vi "ProgressBar-Reset specific progress bar.vi"(8 "Error in":errorcluster, 10 "Sender":enum16{"Acquisition", "Logging", "File gen"}(ring), 11 "Z-stack queue cluster":T1={"Imaging Protocol"=enum."Live Imaging", "Number of Trials"=0, "Frame Size"=512, "# Averaged frames"=0, "Dwell time (us)"=0.0, "Index of Z-plane"=0, "Timelapse?"=FALSE, "Logging process is active"=FALSE, "Speed logging enabled"=FALSE, "tdms file ref"=refnum, "path"=path "", "Trial Number"=0, "Expected # points acquired"=FALSE, "Manually stopped"=FALSE, "Ch0 data"=[], "Ch1 data"=[], "Ref Data"=[], "Last trial"=FALSE, "Ref Dwell time (us)"=0.0, "# Ref Averaged frames"=0, "Ref X Length"=0, "Ref Y Length"=0, "Points acquired"={"Ch0 last trial"=0, "Ch1 last trial"=0, "All trials"=0}} {"Ref Dwell time (us)" format="%#.6g"; "Frame Size" items=["100X100"=100, "128X128"=128, "200X200"=200, "256X256"=256, "512X512"=512, "1024x1024"=1024, "2048x2048"=2048]; "Dwell time (us)" format="%#.6g"}) -> (0 "error out":errorcluster)   [LabVIEW 2017]
uses:
  Typedefs/Logging queue element.ctl
  Typedefs/Imaging Protocols enum.ctl
  Typedefs/Frame Size.ctl
  Typedefs/Acquired points count.ctl
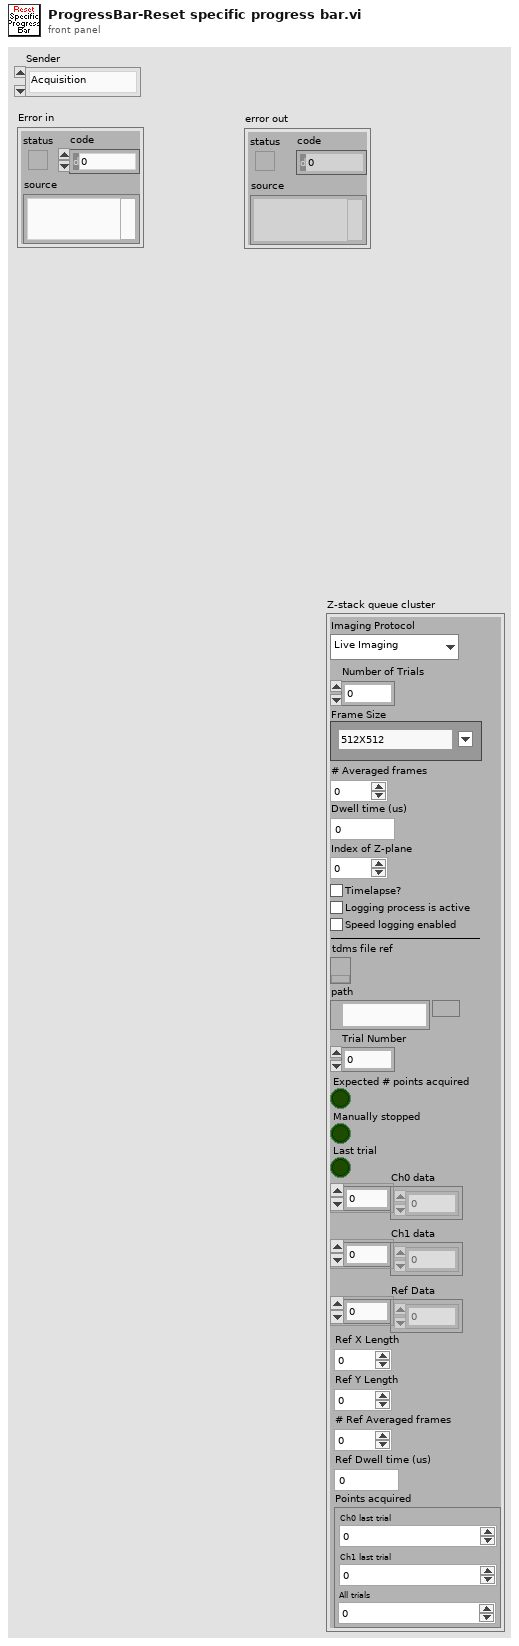
[diagram p1: front panel]
types:
  T1 = typedef "Logging queue element.ctl" = cluster{"Imaging Protocol":T2, "Number of Trials":u16, "Frame Size":T3, "# Averaged frames":u16, "Dwell time (us)":dbl, "Index of Z-plane":i32, "Timelapse?":bool, "Logging process is active":bool, "Speed logging enabled":bool, "tdms file ref":refnum<k34>, "path":path, "Trial Number":i32, "Expected # points acquired":bool, "Manually stopped":bool, "Ch0 data":u32[], "Ch1 data":u32[], "Ref Data":u32[], "Last trial":bool, "Ref Dwell time (us)":dbl, "# Ref Averaged frames":u16, "Ref X Length":u16, "Ref Y Length":u16, "Points acquired":T4}
  T2 = typedef "Imaging Protocols enum.ctl" = enum16{"AOL Z-Stack", "Motor Z Stack", "Functional Acquisition", "Single Plane Acquisition", "Volume Acquisition", "Live Imaging", "Live Plane Imaging", "Live Volume Imaging"}
  T3 = typedef "Frame Size.ctl" = u16
  T4 = typedef "Acquired points count.ctl" = cluster{"Ch0 last trial":u64, "Ch1 last trial":u64, "All trials":u64}
  T5 = typedef "Progress bar window values input cluster.ctl" = cluster{"Total":i32, "Current":i32, "Message in":string, "Sender":enum16{"Acquisition", "Logging", "File gen"}}
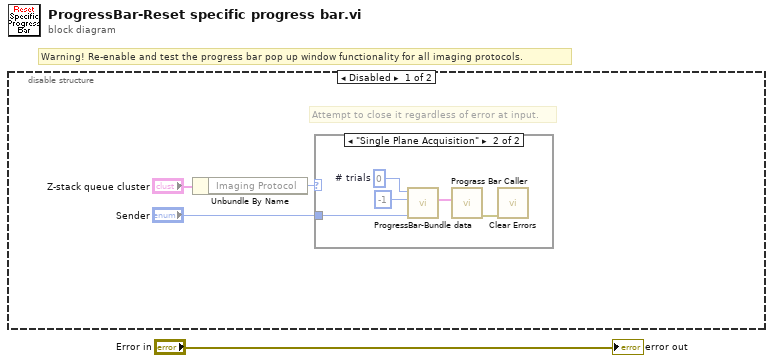
[diagram p0: block diagram]
diagram:
  # "Warning! Re-enable and test the progress bar pop up window functionality for all imaging protocols."
  n1 = disable-structure shown="Disabled" {
    frame Disabled {
      # "Attempt to close it regardless of error at input."
      n2 = Unbundle By Name("Z-stack queue cluster") -> ("Imaging Protocol"=w2:T2)
      n3 = case shown="\"Single Plane Acquisition\"" w2 {
        tunnel: "Sender" -> [_ w7]
        frame "Live Imaging", Default {
        }
        frame "Single Plane Acquisition" {
          w6 = 0  # # trials
          n4 = call "ProgressBar-Bundle data.vi"("Sender"=w7, "Current"=-1, "Total"=w6) -> ("Progress bar window values input"=w8:T5)  [unwired: 8 in]
          n5 = call "Prograss Bar Caller.vi"("Progress bar window values input"=w8) -> ("error out"=w5:errorcluster)  [unwired: 10 in]
          n6 = call <vilib>:"Clear Errors.vi"("error in (no error)"=w5) -> ()  [unwired: 6 in, 1 out]
        }
      }
    }
    frame Enabled {
    }
  }
  "error out" <- "Error in"
